vi "Motor Position Control.vi"() -> ()   [LabVIEW 2013]
uses:
  SGDV_Driver/SGDV_Ctrl_v13_lib/Controls and General VIs/Motor IO Refnum.ctl
  <vilib>/myRIO/Common/Instrument Driver Framework/Utilities/typedefs/Generic FPGA Reference.ctl
  SGDV_Driver/SGDV_Ctrl_v13_lib/Controls and General VIs/Servo Drive and  Motor Paras.ctl
  SGDV_Driver/SGDV_Ctrl_v13_lib/Controls and General VIs/Pos Ctrl Paras.ctl
  SGDV_Driver/SGDV_Ctrl_v13_lib/Controls and General VIs/PID Paras.ctl
  SGDV_Driver/SGDV_Ctrl_v13_lib/Controls and General VIs/Init Motor Data.ctl
  SGDV_Driver/SGDV_Ctrl_v13_lib/SGDV_Ctrl_Class/SGDV_Ctrl_Class.lvclass
  SGDV_Driver/SGDV_Ctrl_v13_lib/SGDV_Ctrl_Class/SGDV_Ctrl_Class.lvclass/SGDV_Ctrl_Class.ctl
  SGDV_Driver/SGDV_Ctrl_v13_lib/SGDV_Ctrl_v13_lib.lvlib
panel:
  in  "Motor Index":u16(ring) items=["Motor 0", "Motor 1", "Motor 2"]
  in  "Motor 2 Refnum":T1={"SEN"="B/AO0", "PWM"="A/PWM2", "SIGN (Vel Dir)"="A/DIO2", "Enc"="C/ENC0", "Generic FPGA Reference"=refnum, "SON"="B/DIO0"}
  in  "Motor 1 Refnum":T1={"SEN"="A/AO1", "PWM"="A/PWM1", "SIGN (Vel Dir)"="A/DIO1", "Enc"="B/ENC", "Generic FPGA Reference"=refnum, "SON"="B/DIO0"}
  out "Pos Curve Set-Current(deg)":cluster{dbl, "Pos Passed(deg)":dbl}(graph)
  out "error out":errorcluster
  in  "Delta Motor Pos(deg)":dbl(slide) scale=-3600.0..3600.0
  in  "stop":bool
  out "Init Motor Data":T3
  in  "error in (no error)":errorcluster
  in  "PID Paras":T4={"Output Range(deg/s)"={"output high"=720.0, "output low"=-720.0}, "PID gains"={"proportional gain (Kc)"=6.5, "integral time (Ti, min)"=0.0075, "derivative time (Td, min)"=0.0005}} {"PID gains"."derivative time (Td, min)" format="%.4f"; "PID gains"."integral time (Ti, min)" format="%.4f"; "PID gains"."proportional gain (Kc)" format="%.4f"; "Output Range(deg/s)"."output low" format="%.2f"; "Output Range(deg/s)"."output high" format="%.2f"}
  in  "Pos Ctrl Paras":T5={"Tolerance(deg)"=0.5, "Loop Time(ms)"=10, "Min Frequency(hz)"=40.0} {"Min Frequency(hz)" format="%#_13g"}
  in  "Servo Drive and  Motor Paras":T6={"Encoder Output Pulses"=900.0, "Gear Ratio(Numerator)"=1000.0, "Gear Ratio(Denominator)"=1.0, "Reduction Ratio"=1.0} {"Gear Ratio(Denominator)" format="%#_10g"}
  in  "Motor IO Refnum":T1={"SEN"="A/AO0", "PWM"="A/PWM0", "SIGN (Vel Dir)"="A/DIO0", "Enc"="A/ENC", "Generic FPGA Reference"=refnum, "SON"="B/DIO0"}
  # "Parameters Setting Before Using SGDV_Ctrl_v13.lvlib.\n1. Set Pn000.1 = 1. (SGDV Control Mode Set: Position Control)\n2. Set Pn50A = 8100, Pn50B = 8848. (SGDV Pin Assignment Set)\n3. Set Pn212 = 900. (SGDV Encoder Pulses Output Set)\n4. Set Pn20E = 1000(Numerator), Pn210 = 1(Denominator). (SGDV Gear Ratio Set)"
  # "(Related to Init Motor Pos.)"
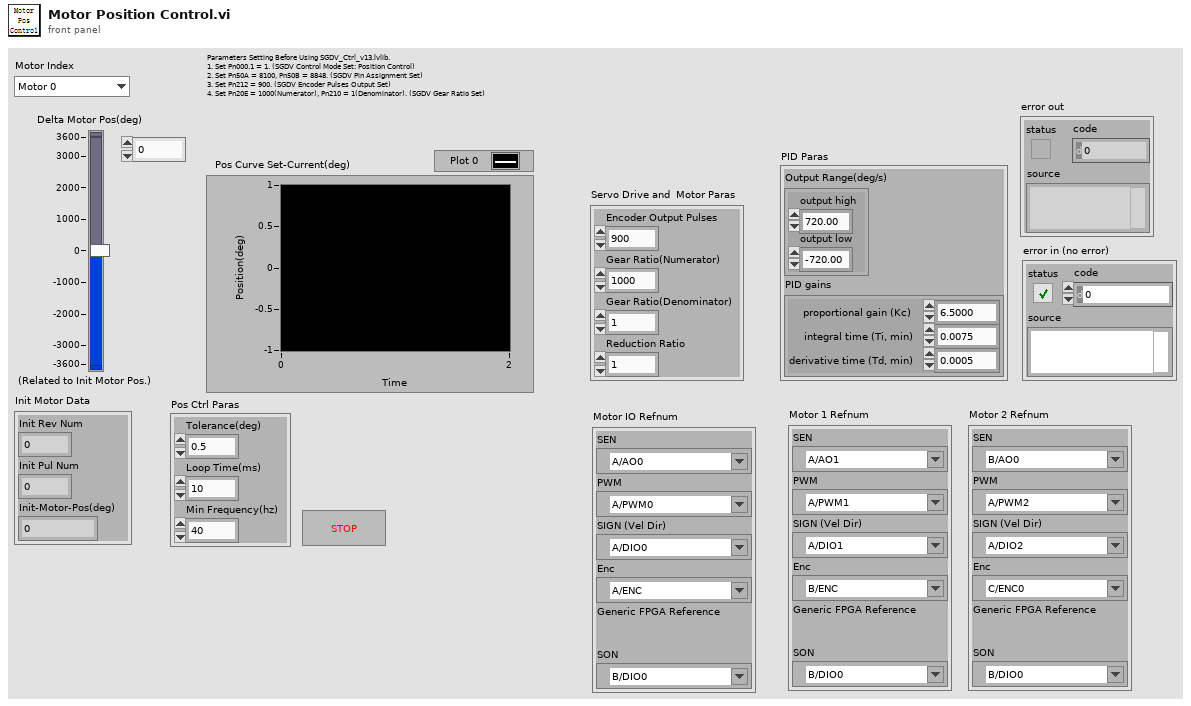
[diagram p1: front panel]
types:
  T1 = typedef "SGDV_Ctrl_v13_lib.lvlib/Motor IO Refnum.ctl" = cluster{"SEN":tag, "PWM":tag, "SIGN (Vel Dir)":tag, "Enc":tag, "Generic FPGA Reference":T2, "SON":tag}
  T2 = typedef "Generic FPGA Reference.ctl" = refnum<k20>
  T3 = typedef "SGDV_Ctrl_v13_lib.lvlib/Init Motor Data.ctl" = cluster{"Init Rev Num":i32, "Init Pul Num":i32, "Init-Motor-Pos(deg)":dbl}
  T4 = typedef "SGDV_Ctrl_v13_lib.lvlib/PID Paras.ctl" = cluster{"Output Range(deg/s)":cluster{"output high":dbl, "output low":dbl}, "PID gains":cluster{"proportional gain (Kc)":dbl, "integral time (Ti, min)":dbl, "derivative time (Td, min)":dbl}}
  T5 = typedef "SGDV_Ctrl_v13_lib.lvlib/Pos Ctrl Paras.ctl" = cluster{"Tolerance(deg)":dbl, "Loop Time(ms)":u32, "Min Frequency(hz)":dbl}
  T6 = typedef "SGDV_Ctrl_v13_lib.lvlib/Servo Drive and  Motor Paras.ctl" = cluster{"Encoder Output Pulses":dbl, "Gear Ratio(Numerator)":dbl, "Gear Ratio(Denominator)":dbl, "Reduction Ratio":dbl}
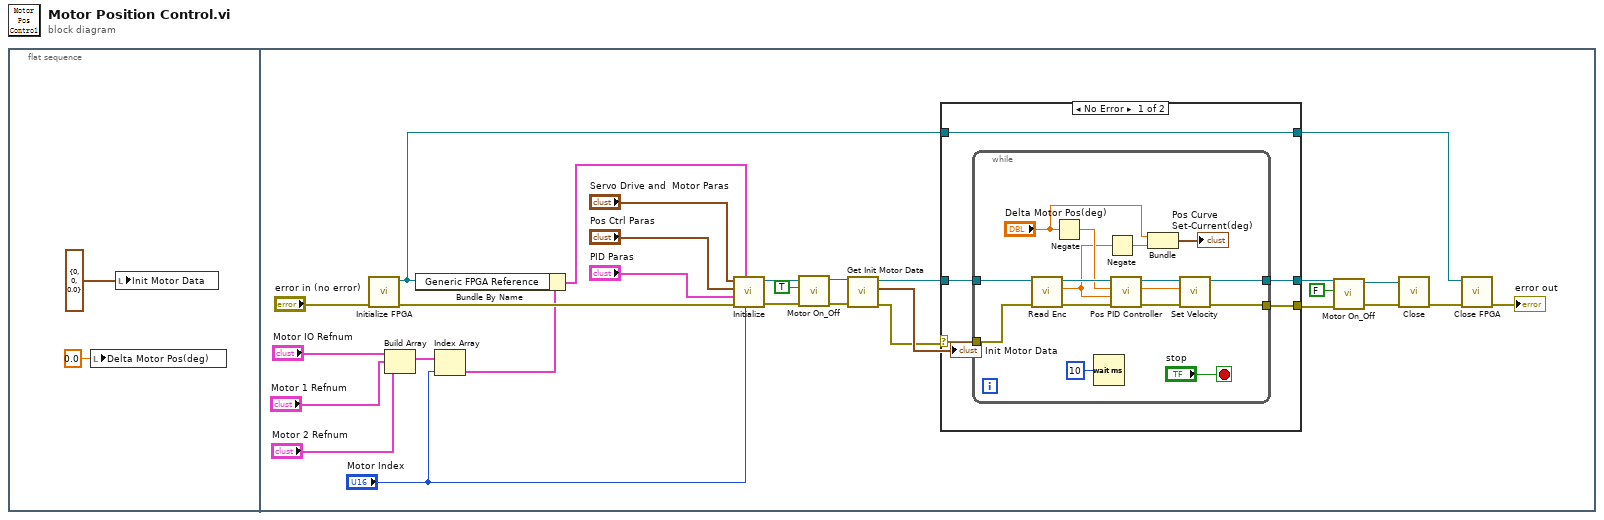
[diagram p0: block diagram]
diagram:
  n1 = flat-sequence {
    frame #0 {
      n2 = local write "Delta Motor Pos(deg)"(0.0 ("Delta Motor Pos(deg)")) -> ()
      n3 = local write "Init Motor Data"(T3 {"Init Rev Num"=0, "Init Pul Num"=0, "Init-Motor-Pos(deg)"=0.0} ("Init Motor Data")) -> ()
    }
    frame #1 {
      n4 = call "Initialize FPGA.vi"("error in (no error)"="error in (no error)") -> ("error out"=w26:errorcluster, "Generic FPGA Reference"=w21:T2)  [unwired: 9 in]
      n5 = Build Array("Motor IO Refnum", "Motor 1 Refnum", "Motor 2 Refnum") -> (w5:T1[])
      n6 = Index Array(array=w5, index="Motor Index") -> (element=w4:T1)
      n7 = Bundle By Name(cluster=w4, "Generic FPGA Reference"=w21) -> (w25:T1)
      n8 = call "Initialize.vi"("Motor Index"="Motor Index", "Motor IO Refnum"=w25, "error in (no error)"=w26, "PID Paras"="PID Paras", "Pos Ctrl Paras"="Pos Ctrl Paras", "Servo Drive and  Motor Paras"="Servo Drive and  Motor Paras") -> ("error out"=w17:errorcluster, "SGDV_Ctrl_Class out"=w18:refnum<class "SGDV_Ctrl_Class.lvclass">)  [unwired: 4 in]
      n9 = call-dynamic "Motor On_Off.vi"("error in (no error)"=w17, "On/Off"=TRUE, "SGDV_Ctrl_Class in"=w18) -> ("error out"=w14:errorcluster, "SGDV_Ctrl_Class out"=w15:refnum<class "SGDV_Ctrl_Class.lvclass">)  [unwired: 7 in]
      n10 = call "Get Init Motor Data.vi"("error in (no error)"=w14, "SGDV_Ctrl_Class in"=w15) -> ("error out"=w23:errorcluster, "Init Motor Data"=→"Init Motor Data":T3, "SGDV_Ctrl_Class out"=w24:refnum<class "SGDV_Ctrl_Class.lvclass">)  [unwired: 7 in]
      n11 = case shown="No Error" w23 {
        selector: w23 -> [w35 w54]
        tunnel: w24 -> [w36 w55]
        tunnel: [w34 w54] -> w13
        tunnel: [w33 w55] -> w10
        tunnel: w21 -> [w32 w53]
        tunnel: [w32 w53] -> w19
        frame No Error {
          n12 = while {
            tunnel: w36 -> [w51]
            tunnel: w35 -> [w44]
            tunnel: [w43] -> w34
            tunnel: [w42] -> w33
            stop <- "stop" stop-if-true
            n13 = call-dynamic "Read Enc.vi"("error in (no error)"=w44, "SGDV_Ctrl_Class in"=w51) -> ("error out"=w46:errorcluster, "Pos Passed(deg)"=w39:dbl, "SGDV_Ctrl_Class out"=w50:refnum<class "SGDV_Ctrl_Class.lvclass">)  [unwired: 7 in]
            n14 = Negate(x="Delta Motor Pos(deg)") -> (-x=w41:dbl)
            n15 = Wait (ms)(milliseconds to wait=u32 10) -> ()  [unwired: 1 out]
            n16 = Negate(x=w39) -> (-x=w38:dbl)
            n17 = call "Pos PID Controller.vi"("error in (no error)"=w46, "Pos Passed(deg)"=w39, "Delta Motor Pos(deg)"=w41, "SGDV_Ctrl_Class in"=w50) -> ("error out"=w45:errorcluster, "Output Vel(deg/s)"=w47:dbl, "SGDV_Ctrl_Class out"=w48:refnum<class "SGDV_Ctrl_Class.lvclass">)  [unwired: 5 in]
            n18 = Bundle("Delta Motor Pos(deg)"="Delta Motor Pos(deg)", w38) -> (→"Pos Curve Set-Current(deg)":cluster{"Delta Motor Pos(deg)":dbl, dbl})  [unwired: 1 in]
            n19 = call "Set Velocity.vi"("error in (no error)"=w45, "Velocity In(deg/s)"=w47, "SGDV_Ctrl_Class in"=w48) -> ("error out"=w43:errorcluster, "SGDV_Ctrl_Class out"=w42:refnum<class "SGDV_Ctrl_Class.lvclass">)  [unwired: 7 in]
          }
        }
        frame Error {
        }
      }
      n20 = call-dynamic "Motor On_Off.vi"("error in (no error)"=w13, "On/Off"=FALSE, "SGDV_Ctrl_Class in"=w10) -> ("error out"=w12:errorcluster, "SGDV_Ctrl_Class out"=w11:refnum<class "SGDV_Ctrl_Class.lvclass">)  [unwired: 7 in]
      n21 = call "Close.vi"("error in (no error)"=w12, "SGDV_Ctrl_Class in"=w11) -> ("error out"=w20:errorcluster)  [unwired: 8 in, 1 out]
      n22 = call "Close FPGA.vi"("error in (no error)"=w20, "Generic FPGA Reference"=w19) -> ("error out"=→"error out":errorcluster)  [unwired: 9 in]
    }
  }
